vi "Personal Information2String.vi"(8 "error in (no error)":errorcluster caption="错误输入（无错误）", 11 "personal information":T1[](array[typedef])) -> (0 "error out":errorcluster caption="错误输出", 3 "personal information":string[][](array[string]))   [LabVIEW 2015, in "Utility VIs.lvlib"]
doc: "该模板用于创建子VI。"
uses:
  Utility VIs.lvlib
  Database Processing/Support/Table/personal_information.ctl
  Database Processing/Database Processing.lvlib
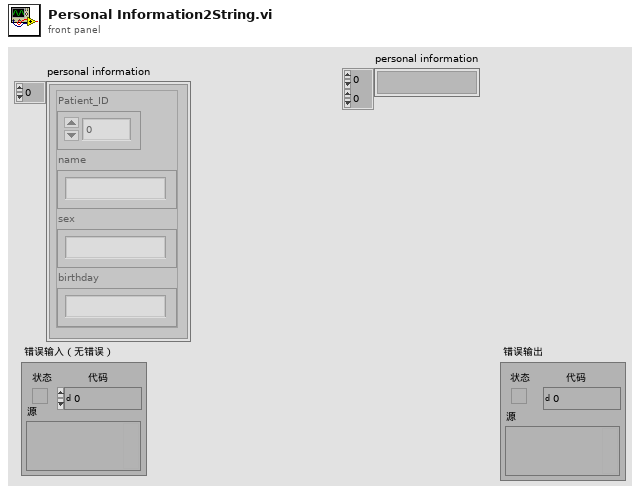
[diagram p1: front panel]
types:
  T1 = typedef "Database Processing.lvlib/personal_information.ctl" = cluster{"Patient_ID":i64, "name":string, "sex":string, "birthday":string}
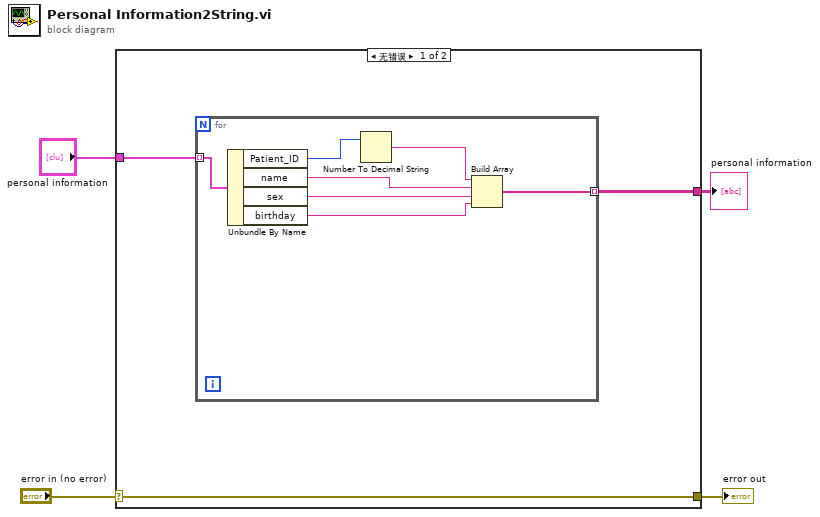
[diagram p0: block diagram]
diagram:
  n1 = case shown="无错误" "error in (no error)" {
    selector: "error in (no error)" -> [w6 w15]
    tunnel: [w6 w15] -> w3
    tunnel: "personal information" -> [w7 _]
    tunnel: [w5 _] -> w1
    frame No Error {
      n2 = for {
        tunnel: w7 -> [w14] mode=indexing
        tunnel: [w8] -> w5 mode=indexing
        n3 = Unbundle By Name(w14) -> ("Patient_ID"=w13:i64, "name"=w11:string, "sex"=w10:string, "birthday"=w9:string)
        n4 = Number To Decimal String(number=w13) -> (decimal integer string=w12:string)  [unwired: 1 in]
        n5 = Build Array(w12, w11, w10, w9) -> (w8:string[])
      }
    }
    frame Error {
    }
  }
  "error out" <- w3
  "personal information" <- w1
